vi "Dispense FN - OFF - Hydration (SubVI).vi"(1 "ON Signal":bool, 2 "Values":T1 {"Time Elapsed (s)" format="%.2f"; "Time Target (s)" format="%.2f"; "Dynamic Setpoint (g)" format="%.2f"; "Static Setpoint (g)" format="%.2f"; "Grams to Setpoint" format="%.2f"; "Adjusted Mass (g)" format="%.2f"; "Dispense Rate (g/sec)" format="%.2f"; "Fill Mass (g)" format="%.2f"; "Fill Rate (g/sec)" format="%.2f"}) -> (0 "Hydration (g)":dbl)   [LabVIEW 2012]
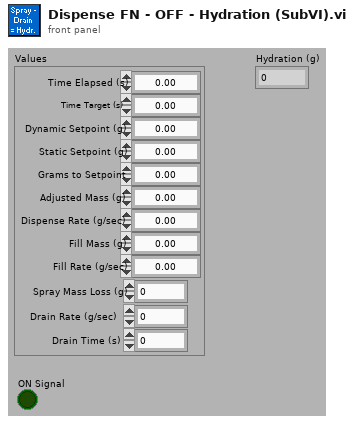
[diagram p1: front panel]
types:
  T1 = cluster{"Time Elapsed (s)":dbl, "Time Target (s)":dbl, "Dynamic Setpoint (g)":dbl, "Static Setpoint (g)":dbl, "Grams to Setpoint":dbl, "Adjusted Mass (g)":dbl, "Dispense Rate (g/sec)":dbl, "Fill Mass (g)":dbl, "Fill Rate (g/sec)":dbl, "Spray Mass Loss (g)":dbl, "Drain Rate (g/sec)":dbl, "Drain Time (s)":dbl}
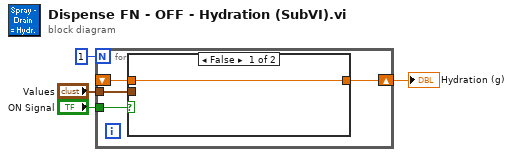
[diagram p0: block diagram]
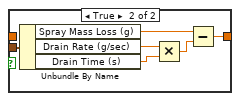
[diagram p2: hidden frame]
diagram:
  n1 = for {
    N: 1 -> [_]
    tunnel: "Values" -> [w8]
    shift-right: [w7] -> w2
    shift-left: _ -> [w6]
    tunnel: "ON Signal" -> [w5]
    n2 = case shown="False" w5 {
      tunnel: w8 -> [_ w15]
      tunnel: [w9 w10] -> w7
      tunnel: w6 -> [w9 _]
      frame False {
      }
      frame True {
        n3 = Unbundle By Name(w15) -> ("Spray Mass Loss (g)"=w12:dbl, "Drain Rate (g/sec)"=w14:dbl, "Drain Time (s)"=w13:dbl)
        n4 = Multiply(x=w14, y=w13) -> (x*y=w11:dbl)
        n5 = Subtract(x=w12, y=w11) -> (x-y=w10:dbl)
      }
    }
  }
  "Hydration (g)" <- w2
